vi "Add.vi"(10 "y":dbl, 11 "x":dbl) -> (2 "x+y":dbl)   [LabVIEW 2019]
panel:
  in  "Boolean":bool
  in  "Numeric":dbl
  out "Waveform Chart":dbl(graph)
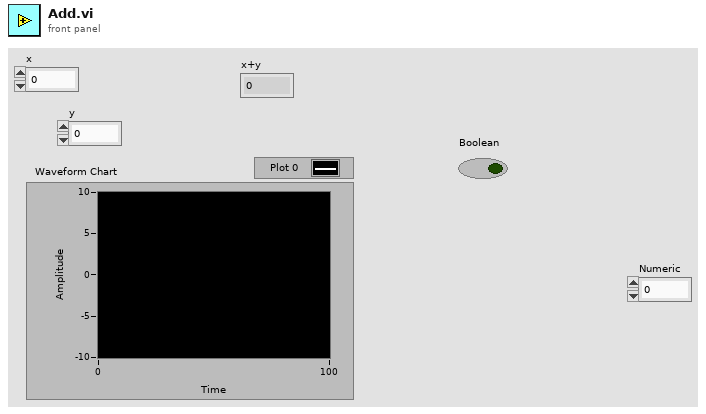
[diagram p1: front panel]
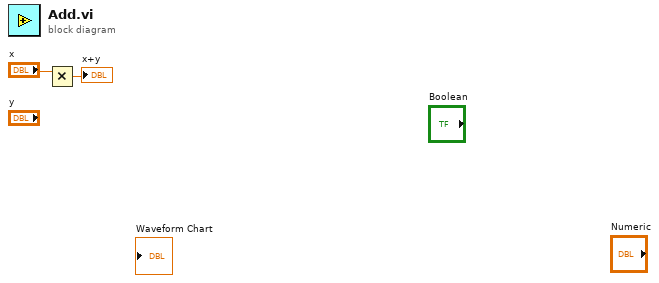
[diagram p0: block diagram]
diagram:
  n1 = Multiply(x="x") -> (x*y=→"x+y":dbl)  [unwired: 1 in]
